vi "CRYOpen Text File.vi"(9 "Index":i32[](array[numeric]), 10 "sOption":string, 11 "File Path":path) -> (2 "Results":T2[](array[typedef]) {"Margin" format="%.2f"}, 3 "Data":T1[](array[typedef]) {"Z data" items=["dB", "Lin"]; "X data" items=["dB", "Lin"]; "Y data" items=["dB", "Lin"]; "Z dB ref" format="%.1f"; "Z axis" items=["Log", "Lin"]; "X dB ref" format="%.1f"; "X axis" items=["Log", "Lin"]; "Y axis" items=["Log", "Lin"]; "Y dB ref" format="%.1f"; "Curve"."z" format="%.2f"; "Curve"."y" format="%.2f"; "Curve"."x" format="%.2f"})   [LabVIEW 2013]
uses:
  CRYSystem/Typedef Control/CRYResult Cluster.ctl
  CRYSystem/Typedef Control/CRYData Cluster.ctl
  CRYSystem/Typedef Control/CRYResult Cluster Array.ctl
  Global/CRYCurve Library Global.vi
panel:
  # "Open All Data(Curves, Values,Results, Waveforms)"
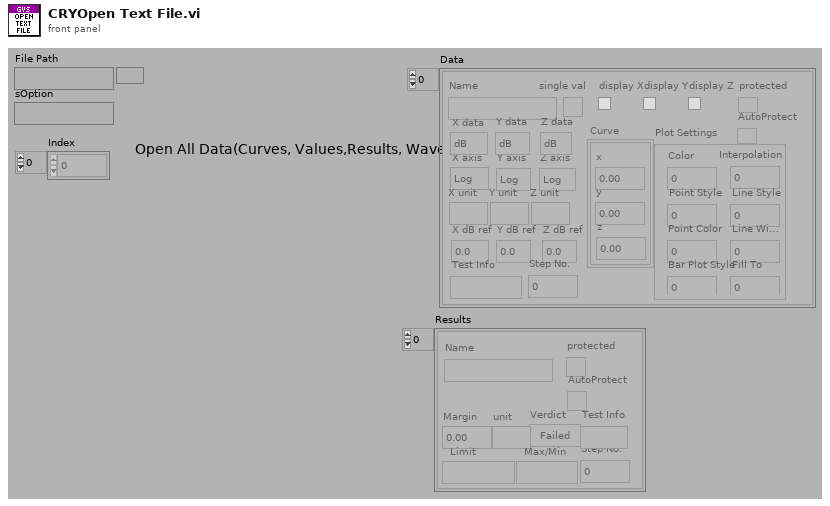
[diagram p1: front panel]
types:
  T1 = typedef "CRYData Cluster.ctl" = cluster{"Name":string, "Curve":cluster{"x":dbl, "y":dbl, "z":dbl}[], "X data":u16, "Y data":u16, "Z data":u16, "X axis":u16, "Y axis":u16, "Z axis":u16, "X unit":string, "Y unit":string, "Z unit":string, "X dB ref":dbl, "Y dB ref":dbl, "Z dB ref":dbl, "single val":bool, "protected":bool, "display X":bool, "display Y":bool, "display Z":bool, "Test Info":string, "Step No.":i32, "Plot Settings":cluster{"Color":u32, "Interpolation":u8, "Point Style":u8, "Line Style":u8, "Point Color":u32, "Line Width":u8, "Bar Plot Style":u8, "Fill To":i16}, "AutoProtect":bool}
  T2 = typedef "CRYResult Cluster.ctl" = cluster{"Name":string, "Margin":dbl, "unit":string, "Verdict":bool, "Limit":string, "Max/Min":string, "protected":bool, "Step No.":i32, "Test Info":string, "AutoProtect":bool}
  T3 = typedef "CRYResult Cluster Array.ctl" = T2[]
  T4 = enum16{"read/write", "read-only", "write-only", "write-only (truncate)"}
  T5 = enum16{"OK", "Yes", "YesNo", "YesNoCancel", "ReplaceAppend"}
  T6 = typedef "CRYData Cluster Array.ctl" = T1[]
  T7 = cluster{"Color":u32, "Interpolation":u8, "Point Style":u8, "Line Style":u8, "Point Color":u32, "Line Width":u8, "Bar Plot Style":u8, "Fill To":i16}
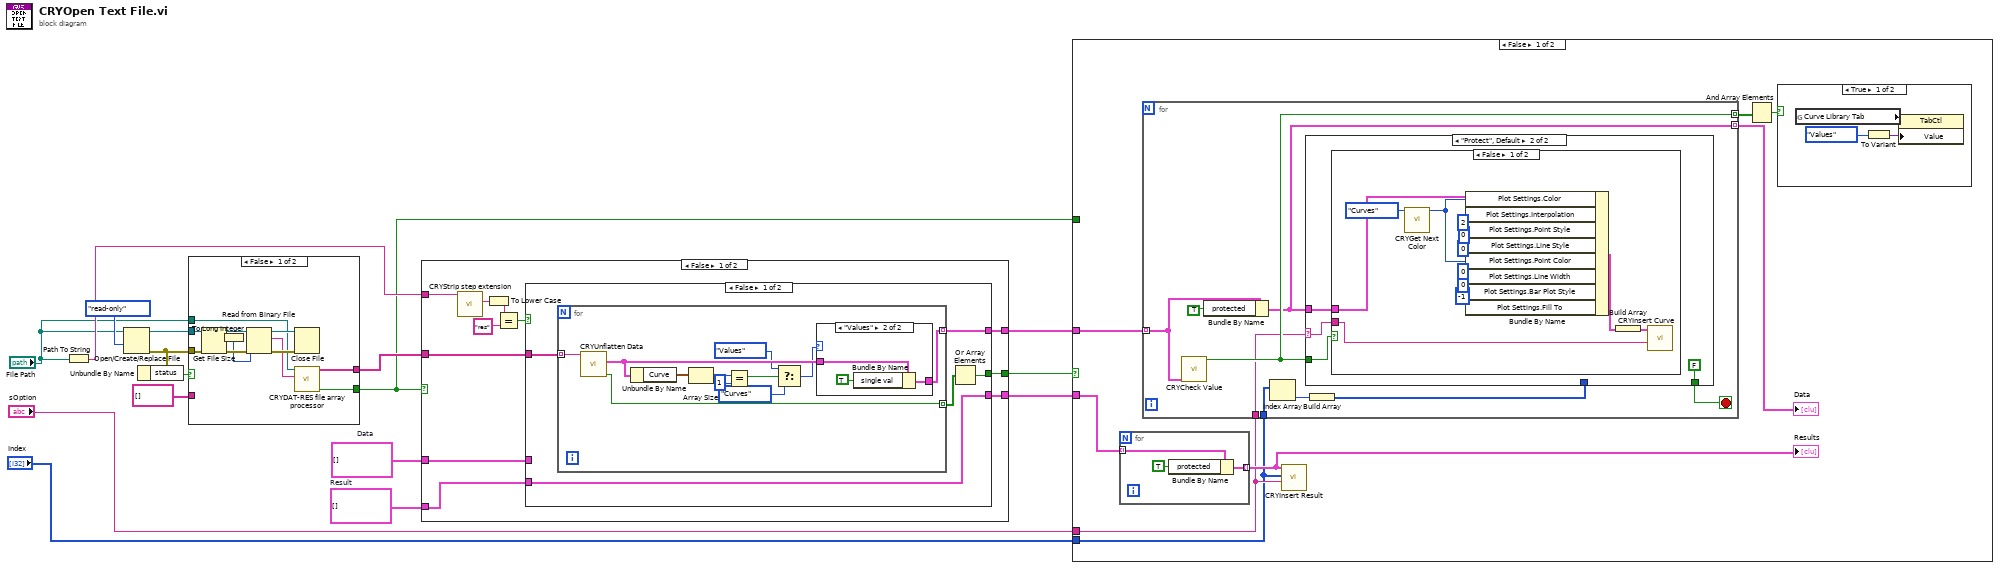
[diagram p0: block diagram]
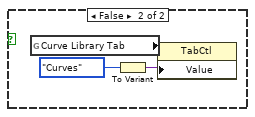
[diagram p2: hidden frame]
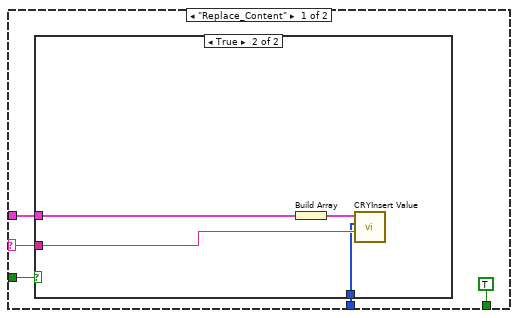
[diagram p3: hidden frame]
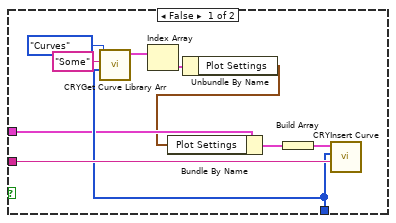
[diagram p4: hidden frame]
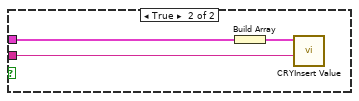
[diagram p5: hidden frame]
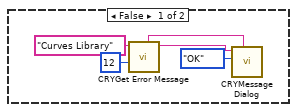
[diagram p7: hidden frame]
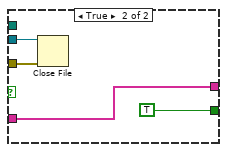
[diagram p8: hidden frame]
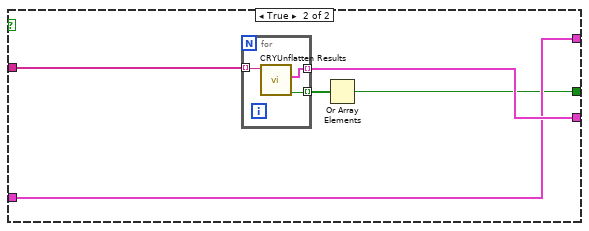
[diagram p10: hidden frame]
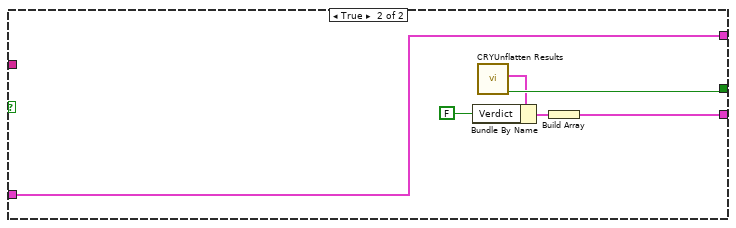
[diagram p11: hidden frame]
diagram:
  w8 = T3 []  # Result
  w15 = T1[] []  # Data
  n1 = Path To String(path="File Path") -> (string=w16:string)
  n2 = Open/Create/Replace File(file path (use dialog)="File Path", access (0:read/write)=T4."read-only" ("open mode (0)")) -> (refnum out=w11:refnum<file>, error out=w12:errorcluster)  [unwired: 1 in, 4 out]
  n3 = Unbundle By Name(w12) -> ("status"=w13:bool)
  n4 = case shown="False" w13 {
    tunnel: w12 -> [w23 w32]
    tunnel: w11 -> [w22 w31]
    tunnel: "File Path" -> [w20 _]
    tunnel: string[] [] ("Data curves array") -> [_ w29]
    tunnel: [w19 w29] -> w9
    tunnel: [w18 TRUE ("Canceled")] -> w1
    frame False {
      n5 = Get File Size(file=w22, error in=w23) -> (refnum out=w25:refnum<file>, size (in bytes)=w17:i64, 0:w26:errorcluster)
      n6 = To Long Integer(number=w17) -> (32bit integer=w24:i32)
      n7 = Read from Binary File(8:w26, 10:w24, 11:w25) -> (0:w28:errorcluster, 2:w21:string, 3:w27:refnum<file>)  [unwired: 4 out]
      n8 = Close File(refnum=w27, error in=w28) -> ()  [unwired: 2 out]
      n9 = call "CRYDAT-RES file array processor.vi"("Entire file contents"=w21, "Filepath"=w20) -> ("Canceled"=w18:bool, "Array of flat Data or Results"=w19:string[])  [unwired: 8 in]
    }
    frame True {
      n10 = Close File(refnum=w31, error in=w32) -> ()  [unwired: 2 out]
    }
  }
  n11 = case shown="False" w1 {
    tunnel: w9 -> [w38 _]
    tunnel: w16 -> [w40 _]
    tunnel: [w37 w77] -> w4
    tunnel: [w36 w75] -> w3
    tunnel: w15 -> [w35 w77]
    tunnel: w8 -> [w34 _]
    tunnel: [w33 w73] -> w2
    frame False {
      n12 = call "CRYStrip step extension.vi"("Step name w/ extension"=w40) -> ("Extension (3-letter category)"=w43:string)  [unwired: 7 in, 3 out]
      n13 = To Lower Case(string=w43) -> (all lower case string=w41:string)
      n14 = Equal?(x=w41, y="res") -> (x = y?=w39:bool)
      n15 = case shown="False" w39 {
        tunnel: w38 -> [w48 w68]
        tunnel: [w47 w66] -> w37
        tunnel: [w46 w67] -> w36
        tunnel: w35 -> [_ w66]
        tunnel: w34 -> [w46 _]
        tunnel: [w44 w64] -> w33
        frame False {
          n16 = for {
            tunnel: w48 -> [w59] mode=indexing
            tunnel: [w58] -> w47 mode=indexing
            tunnel: [w57] -> w45 mode=indexing
            n17 = call "CRYUnflatten Data.vi"("Unflatten data"=w59) -> ("Error?"=w57:bool, "Datum"=w56:T1)  [unwired: 8 in, 1 out]
            n18 = Unbundle By Name(w56) -> ("Curve"=w50:cluster{"x":dbl, "y":dbl, "z":dbl}[])
            n19 = Array Size(array=w50) -> (size(s)=w55:i32)
            n20 = Equal?(x=w55, y=1) -> (x = y?=w53:bool)
            n21 = Select(t=enum16{"Curves", "Values", "Results", "WFM"}."Values" ("Type"), s=w53, f=enum16{"Curves", "Values", "Results", "WFM"}."Curves" ("Type")) -> (s? t:f=w51:enum16{"Curves", "Values", "Results", "WFM"})
            n22 = case shown="\"Values\"" w51 {
              tunnel: w56 -> [w60 w62]
              tunnel: [w60 w61] -> w58
              frame "Curves", Default {
              }
              frame "Values" {
                n23 = Bundle By Name(cluster=w62, "single val"=TRUE ("protected")) -> (w61:T1)
              }
            }
          }
          n24 = Or Array Elements(Boolean array=w45) -> (logical OR=w44:bool)
        }
        frame True {
          n25 = for {
            tunnel: w68 -> [w71] mode=indexing
            tunnel: [w69] -> w67 mode=indexing
            tunnel: [w70] -> w65 mode=indexing
            n26 = call "CRYUnflatten Results.vi"("Unflatten Result"=w71) -> ("Error?"=w70:bool, "Result"=w69:T2)  [unwired: 8 in, 1 out]
          }
          n27 = Or Array Elements(Boolean array=w65) -> (logical OR=w64:bool)
        }
      }
    }
    frame True {
      n28 = call "CRYUnflatten Results.vi"() -> ("Error?"=w73:bool, "Result"=w72:T2)  [unwired: 9 in, 1 out]
      n29 = Bundle By Name(cluster=w72, "Verdict"=FALSE) -> (w74:T2)
      n30 = Build Array(w74) -> (w75:T2[])
    }
  }
  n31 = case shown="False" w2 {
    tunnel: "sOption" -> [w82 _]
    tunnel: "Index" -> [w81 _]
    tunnel: w4 -> [w79 _]
    tunnel: w3 -> [w78 _]
    tunnel: w1 -> [_ w142]
    frame False {
      n32 = for {
        tunnel: w78 -> [w87] mode=indexing
        tunnel: [w86] -> w83 mode=indexing
        n33 = Bundle By Name(cluster=w87, "protected"=TRUE) -> (w86:T2)
      }
      "Results" <- w83
      n34 = for {
        tunnel: w79 -> [w103] mode=indexing
        tunnel: [w102] -> w84 mode=indexing
        tunnel: w82 -> [w100]
        tunnel: w81 -> [w99]
        tunnel: [w95] -> w80 mode=indexing
        stop <- w96 stop-if-true
        n35 = call "CRYCheck Value.vi"("Data"=w103) -> ("Single?"=w102:bool)  [unwired: 2 in, 8 out]
        n36 = Bundle By Name(cluster=w103, "protected"=TRUE) -> (w95:T1)
        n37 = Index Array(array=w99) -> (element=w98:i32)  [unwired: 1 in]
        n38 = Build Array(w98) -> (w97:i32[])
        n39 = case shown="\"Protect\", Default" w100 {
          selector: w100 -> [w106 w124]
          tunnel: w95 -> [w108 w126]
          tunnel: w102 -> [w107 w125]
          tunnel: w97 -> [w105 _]
          tunnel: [TRUE FALSE] -> w96
          frame "Replace_Content" {
            n40 = case shown="True" w107 {
              tunnel: w108 -> [w111 w122]
              tunnel: w106 -> [w117 w120]
              tunnel: w105 -> [w114 w119]
              frame False {
                n41 = call "CRYGet Curve Library Arr.vi"("Index"=w114, "sOption"="Some", "Type In"=enum16{"Curves", "Values", "Results", "WFM"}."Curves") -> ("Curves/Values"=w113:T6)  [unwired: 6 in, 2 out]
                n42 = Index Array(array=w113) -> (element=w112:T1)  [unwired: 1 in]
                n43 = Unbundle By Name(w112) -> ("Plot Settings"=w110:T7)
                n44 = Bundle By Name(cluster=w111, "Plot Settings"=w110) -> (w109:T1)
                n45 = Build Array(w109) -> (w118:T1[])
                n46 = call "CRYInsert Curve.vi"("sOption"=w117, "Index"=w114, "Curve"=w118) -> ()  [unwired: 1 in, 8 out]
              }
              frame True {
                n47 = Build Array(w122) -> (w121:T1[])
                n48 = call "CRYInsert Value.vi"("sOption"=w120, "Index"=w119, "Value"=w121) -> ()  [unwired: 1 in, 8 out]
              }
            }
          }
          frame "Protect", Default {
            n49 = case shown="False" w125 {
              tunnel: w126 -> [w129 w141]
              tunnel: w124 -> [w137 w139]
              frame False {
                n50 = call "CRYGet Next Color.vi"("Type"=enum16{"Curves", "Values", "Results", "WFM"}."Curves") -> ("Color"=w133:u32)  [unwired: 10 out]
                n51 = Bundle By Name(cluster=w129, "Plot Settings.Color"=w133, "Plot Settings.Interpolation"=u8 2, "Plot Settings.Point Style"=u8 0, "Plot Settings.Line Style"=u8 0, "Plot Settings.Point Color"=w133, "Plot Settings.Line Width"=u8 0, "Plot Settings.Bar Plot Style"=u8 0, "Plot Settings.Fill To"=i16 -1) -> (w128:T1)
                n52 = Build Array(w128) -> (w138:T1[])
                n53 = call "CRYInsert Curve.vi"("sOption"=w137, "Curve"=w138) -> ()  [unwired: 2 in, 8 out]
              }
              frame True {
                n54 = Build Array(w141) -> (w140:T1[])
                n55 = call "CRYInsert Value.vi"("sOption"=w139, "Value"=w140) -> ()  [unwired: 2 in, 8 out]
              }
            }
          }
        }
      }
      "Data" <- w80
      n56 = call "CRYInsert Result.vi"("sOption"=w82, "Index"=w81, "Result"=w83) -> ()  [unwired: 7 in, 2 out]
      n57 = And Array Elements(Boolean array=w84) -> (logical AND=w85:bool)
      n58 = case shown="True" w85 {
        frame True {
          n59 = global read "CRYCurve Library Global.vi" "Curve Library Tab"() -> (w91:refnum<vi>)
          n60 = To Variant(anything=enum32{"Curves", "Values", "Results", "WFM"}."Values" ("Value")) -> (Variant=w89:variant)
          n61 = property class="TabCtl"(reference=w91, "Value"=w89) -> ()  [unwired: 1 in, 2 out]
        }
        frame False {
          n62 = global read "CRYCurve Library Global.vi" "Curve Library Tab"() -> (w94:refnum<vi>)
          n63 = To Variant(anything=enum32{"Curves", "Values", "Results", "WFM"}."Curves" ("Value")) -> (Variant=w92:variant)
          n64 = property class="TabCtl"(reference=w94, "Value"=w92) -> ()  [unwired: 1 in, 2 out]
        }
      }
    }
    frame True {
      n65 = case shown="True" w142 {
        frame False {
          n66 = call "CRYGet Error Message.vi"("Error No"=12, "Kind"="Curves Library") -> ("Message"=w144:string, "Window Title"=w143:string)  [unwired: 4 in, 4 out]
          n67 = call "CRYMessage Dialog.vi"("Window Title"=w143, "YesNoCancel"=T5."OK", "Message Content"=w144) -> ()  [unwired: 7 in, 2 out]
        }
        frame True {
          # "in the case of Cancel"
        }
      }
    }
  }
